vi "Path.vi"(8 "Error In":errorcluster, 11 "Queue in":refnum<queue>) -> (0 "Error Out":errorcluster, 3 "Output Path":path)   [LabVIEW 2021, in "Main.lvlib" / "Main_Programs_SubVIs.lvlib"]
doc: "This subVI is used for the operation of file picking."
uses:
  Main_Programs_SubVIs.lvlib
  Tipski Definicii/Save_Sostojbi.ctl
  Polymorphic/Enq_Save_QMH.vi
  Polymorphic/Queues.lvlib
panel:
  # "Input"
  # "Output"
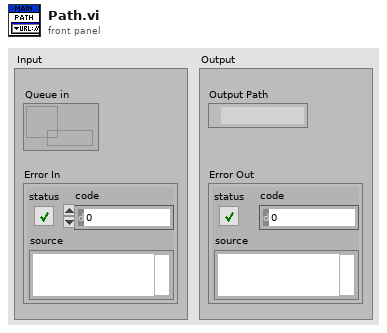
[diagram p1: front panel]
types:
  T1 = typedef "Save_Sostojbi.ctl" = enum16{"Init", "Generate Message", "Pick Path", "Save", "End"}
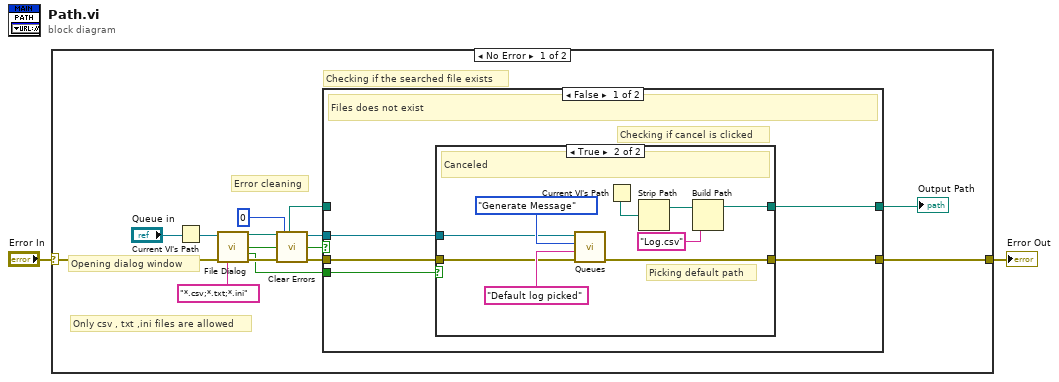
[diagram p0: block diagram]
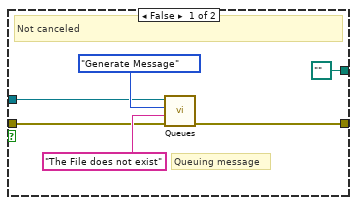
[diagram p2: hidden frame]
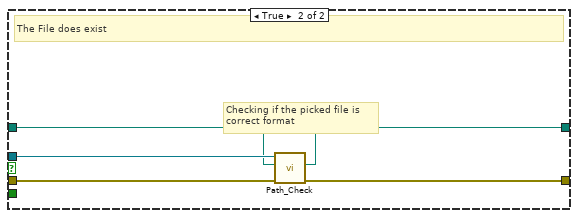
[diagram p3: hidden frame]
diagram:
  n1 = case shown="No Error" "Error In" {
    selector: "Error In" -> [w10 w40]
    tunnel: [w4 w40] -> w1
    frame No Error {
      # "Error cleaning"
      # "Checking if the searched file exists"
      # "Only csv , txt ,ini files are allowed"
      # "Opening dialog window"
      n2 = Current VI's Path() -> (path=w9:path)
      n3 = call "File Dialog"("start path"=w9, "error in"=w10, "pattern (all files)"="*.csv;*.txt;*.ini") -> ("selected path"=w14:path, "exists"=w11:bool, "cancelled"=w5:bool, "error out"=w8:errorcluster)  [unwired: 9 in]
      n4 = call <vilib>:"Clear Errors.vi"("error in (no error)"=w8, "specific error code to clear (0: all)"=0) -> ("error out"=w7:errorcluster)  [unwired: 4 in, 1 out]
      n5 = case shown="False" w11 {
        tunnel: w7 -> [w16 w39]
        tunnel: "Queue in" -> [w15 w38]
        tunnel: [w18 w36] -> w4
        tunnel: w14 -> [_ w37]
        tunnel: [w17 w35] -> w6
        tunnel: w5 -> [w19 _]
        frame False {
          # "Checking if cancel is clicked"
          # "Files does not exist"
          n6 = case shown="True" w19 {
            tunnel: [path "" ("appended path") w32] -> w17
            tunnel: [w22 w29] -> w18
            tunnel: w16 -> [w23 w28]
            tunnel: w15 -> [w21 w27]
            frame False {
              # "Queuing message"
              # "Not canceled"
              n7 = call-poly "Queues.vi"("Error In"=w23, "Message"="The File does not exist", "Instruction"=Save_Sostojbi."Generate Message", "Queue In"=w21) -> ("Error Out"=w22:errorcluster)  [unwired: 6 in, 1 out]
            }
            frame True {
              # "Picking default path"
              # "Canceled"
              n8 = call-poly "Queues.vi"("Error In"=w28, "Message"="Default log picked", "Instruction"=Save_Sostojbi."Generate Message", "Queue In"=w27) -> ("Error Out"=w29:errorcluster)  [unwired: 6 in, 1 out]
              n9 = Current VI's Path() -> (path=w26:path)
              n10 = Strip Path(path=w26) -> (stripped path=w34:path)  [unwired: 1 out]
              n11 = Build Path(base path=w34, name or relative path="Log.csv") -> (appended path=w32:path)
            }
          }
        }
        frame True {
          # "Checking if the picked file is \ncorrect format"
          # "The File does exist"
          n12 = call "Path_Check.vi"("Error In"=w39, "Path In"=w37, "Queue In"=w38) -> ("Error Out"=w36:errorcluster, "Path Out"=w35:path)  [unwired: 6 in, 1 out]
        }
      }
      "Output Path" <- w6
    }
    frame Error {
    }
  }
  "Error Out" <- w1
